vi "semaphore.vi"() -> ()   [LabVIEW 2017]
panel:
  in  "Tab Control":enum32{"Page 1", "Page 2"}(tab)
  in  "?":bool
  in  "Array":cluster{"Boolean":bool, "pin":dbl}[](array[cluster])
  in  "stop":bool
  out "concatenated string":string
  in  "GPIO":string(combo)
  out "Numeric":dbl
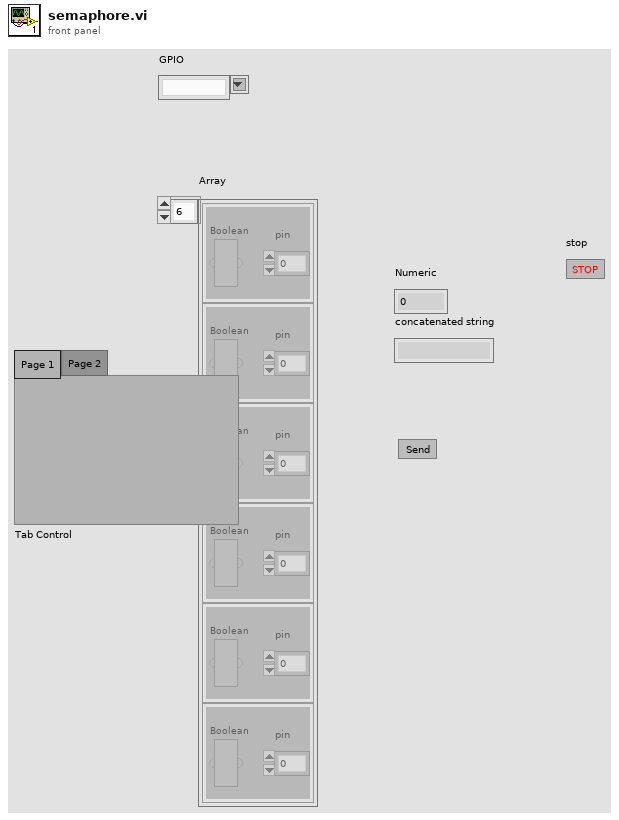
[diagram p1: front panel]
types:
  T1 = typedef "Semaphore RefNum" = refnum<k1>
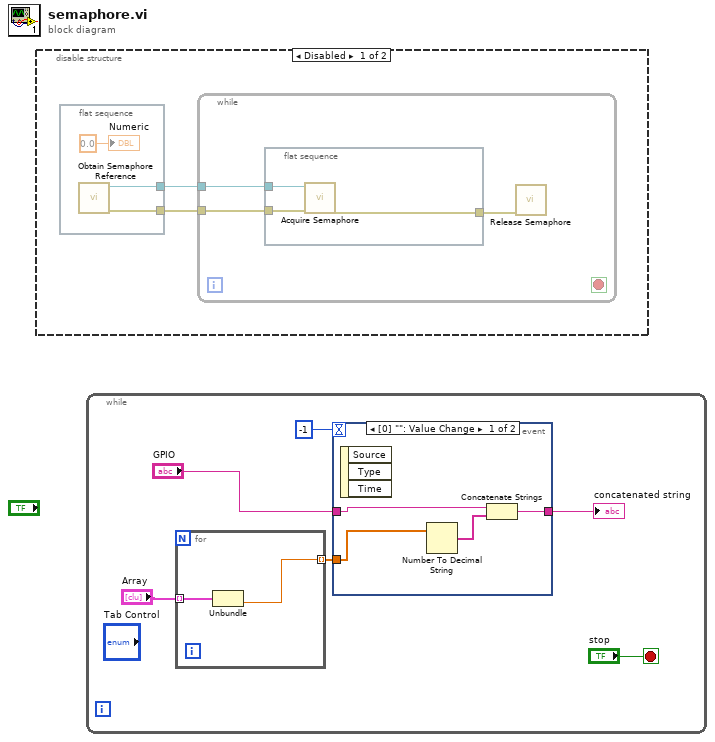
[diagram p0: block diagram]
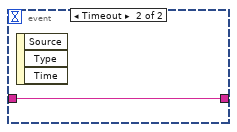
[diagram p2: hidden frame]
diagram:
  n1 = disable-structure shown="Disabled" {
    frame Disabled {
      n2 = flat-sequence {
        tunnel: [w10] -> w2
        tunnel: [w9] -> w1
        frame #0 {
          n3 = call <vilib>:"Obtain Semaphore Reference.vi"() -> ("error out"=w10:errorcluster, "semaphore"=w9:T1)  [unwired: 5 in, 1 out]
          "Numeric" <- 0.0
        }
      }
      n4 = while {
        tunnel: w2 -> [w5]
        tunnel: w1 -> [w3]
        stop <- _ stop-if-true
        n5 = flat-sequence {
          tunnel: w5 -> [w8]
          tunnel: [w7] -> w4
          tunnel: w3 -> [w6]
          frame #0 {
            n6 = call <vilib>:"Acquire Semaphore.vi"("error in (no error)"=w8, "semaphore"=w6) -> ("error out"=w7:errorcluster)  [unwired: 3 in, 2 out]
          }
        }
        n7 = call <vilib>:"Release Semaphore.vi"("error in (no error)"=w4) -> ()  [unwired: 5 in, 2 out]
      }
    }
    frame Enabled {
    }
  }
  n8 = while {
    stop <- "stop" stop-if-true
    n9 = for {
      tunnel: "Array" -> [w24] mode=indexing
      tunnel: [w23] -> w12 mode=indexing
      n10 = Unbundle(w24) -> ("pin"=w23:dbl)  [unwired: 1 out]
    }
    n11 = event shown="[0] \"\": Value Change" {
      selector: _ -> [_ _]
      dyn-events: _ -> [_ _]
      timeout: -1 -> [_ _]
      tunnel: [w20 w22] -> w14
      tunnel: "GPIO" -> [w19 w22]
      tunnel: w12 -> [w18 _]
      event Value Change {
        n12 = event-data() -> ()  [unwired: 1 in, 3 out]
        n13 = Number To Decimal String(number=w18) -> (decimal integer string=w21:string[])  [unwired: 1 in]
        n14 = Concatenate Strings(w19, w21) -> (w20:string)
      }
      event Timeout {
        n15 = event-data() -> ()  [unwired: 1 in, 3 out]
      }
    }
    "concatenated string" <- w14
  }
